vi "Write UI Event.vi"(8 "error in (no error)":errorcluster, 10 "UI Event":refnum<user-event>, 11 "Tasks in":refnum<class "Tasks.lvclass">) -> (0 "error out":errorcluster, 3 "Tasks out":refnum<class "Tasks.lvclass">)   [LabVIEW 2012, in "Tasks.lvclass"]
uses:
  Tasks.lvclass
  Type Defs/Mode Select.ctl
  Tasks.lvclass/Tasks.ctl
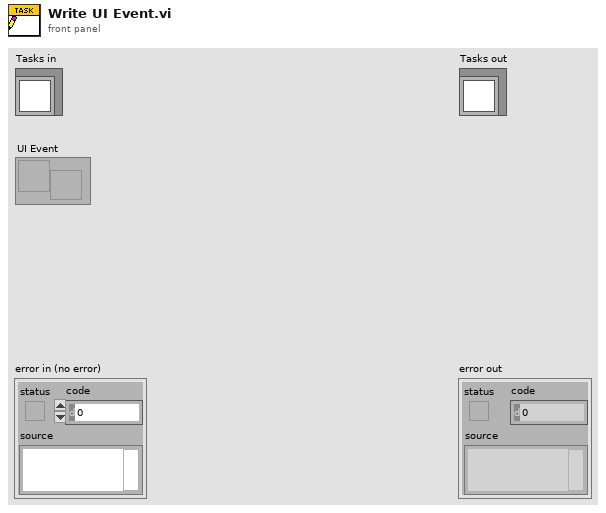
[diagram p1: front panel]
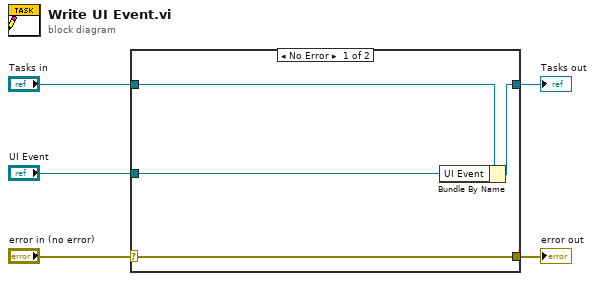
[diagram p0: block diagram]
diagram:
  n1 = case shown="No Error" "error in (no error)" {
    selector: "error in (no error)" -> [w9 w10]
    tunnel: [w9 w10] -> w4
    tunnel: [w7 w11] -> w2
    tunnel: "Tasks in" -> [w8 w11]
    tunnel: "UI Event" -> [w6 _]
    frame No Error {
      n2 = Bundle By Name(cluster=w8, "UI Event"=w6) -> (w7:refnum<class "Tasks.lvclass">)
    }
    frame Error {
    }
  }
  "error out" <- w4
  "Tasks out" <- w2
